vi "LabView - LineFollower.vi"() -> ()   [LabVIEW 2022 SP3]
uses:
  <vilib>/MakerHub/LINX/Public/Peripherals/Digital/Digital Read N Chans.vi
  <vilib>/MakerHub/LINX/Public/Peripherals/Digital/Digital Write N Chans.vi
  <vilib>/MakerHub/LINX/Private/Local IO/LinxDigitalRead.vi
  <vilib>/MakerHub/LINX/Public/Utilities/Check Channel.vi
  <vilib>/MakerHub/LINX/Private/Local IO/LinxDigitalWrite.vi
  <vilib>/MakerHub/LINX/Public/Utilities/Open Serial.vi
  <vilib>/MakerHub/LINX/Private/Utilties/Generate Error.vi
  <vilib>/MakerHub/LINX/Public/Peripherals/PWM/PWM Set Duty Cycle N Chans.vi
  <vilib>/MakerHub/LINX/LMH-LINX.lvlib
panel:
  in  "Slider_Case7":dbl(slide) scale=0.0..1.0
  in  "Slider_Case6":dbl(slide) scale=0.0..1.0
  in  "Slider_Case5":dbl(slide) scale=0.0..1.0
  in  "Slider_Case4":dbl(slide) scale=0.0..1.0
  in  "Slider_Case3":dbl(slide) scale=0.0..1.0
  in  "Slider_Case1":dbl(slide) scale=0.0..1.0
  in  "Slider_Case0":dbl(slide) scale=0.0..1.0
  in  "Array_Case7":bool[](array[boolean])
  in  "Array_Case6":bool[](array[boolean])
  in  "Array_Case5":bool[](array[boolean])
  in  "Array_Case4":bool[](array[boolean])
  in  "ArrayArray_Case3":bool[](array[boolean])
  in  "Array_Case2":bool[](array[boolean])
  in  "Array_Case1":bool[](array[boolean])
  in  "Array_Case0":bool[](array[boolean])
  in  "Motor 1":dbl[](array[slide]) scale=0.0..1.0
  in  "DI Channels":u8[](array[numeric])
  in  "PWM Channels":u8[](array[numeric])
  in  "DO Motor Channels":u8[](array[numeric])
  in  "millisecond timer value":u32
  out "number":u32
  out "String":string
  out "Boolean 2":bool
  out "IR LED":bool[](array[boolean])
  in  "stop":bool
  in  "Serial Port":refnum<visa-resource-name>="N/A"
  # "Motor's PWM"
  # "Motor 1"
  # "Motor 2"
  # "Channels Data"
  # "Data Unit"
  # "IR Cases"
  # "IR Cases Motor's Speed"
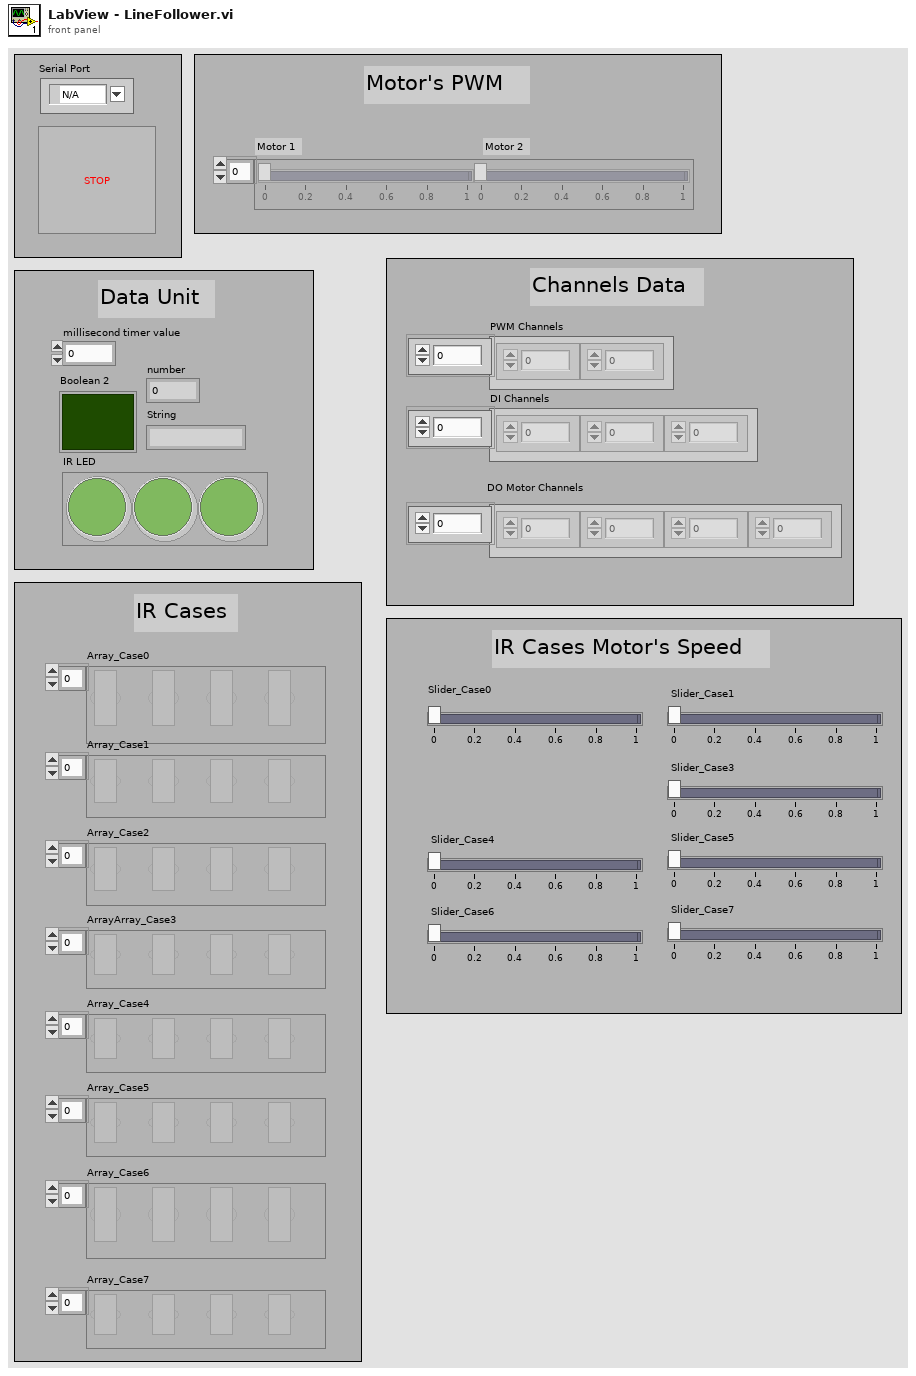
[diagram p1: front panel]
types:
  T1 = typedef "LMH-LINX.lvlib/LINX Ref.ctl" = cluster{"IO":T2, "Interface":T3, "LINX Device Config":T4}
  T2 = typedef "LMH-LINX.lvlib/Platform.ctl" = enum16{"Remote", "Local"}
  T3 = typedef "LMH-LINX.lvlib/Interface.ctl" = enum16{"Serial", "TCP"}
  T4 = typedef "LMH-LINX.lvlib/Device.lvlib/LINX Device Config.ctl" = cluster{"Interface":T3, "COM Port":refnum<visa-resource-name>, "TCP Configuration":T5, "Device Family":u8, "Device ID":u8, "Device Name":string, "TCP Ref":refnum<k5>, "Channels":T6}
  T5 = typedef "LMH-LINX.lvlib/Device.lvlib/TCP Config.ctl" = cluster{"IP Address":string, "Port":u16}
  T6 = typedef "LMH-LINX.lvlib/Channels.ctl" = cluster{"DI":u8[], "DO":u8[], "AI":u8[], "AO":u8[], "PWM":u8[], "QE":u8[], "UART":u8[], "I2C 2":u8[], "SPI":u8[], "CAN":u8[], "Servo":u8[], "AI Ref (V)":dbl, "AI Resolution (Bits)":u8, "AO Ref (V)":dbl, "AO Resolution (Bits)":u8}
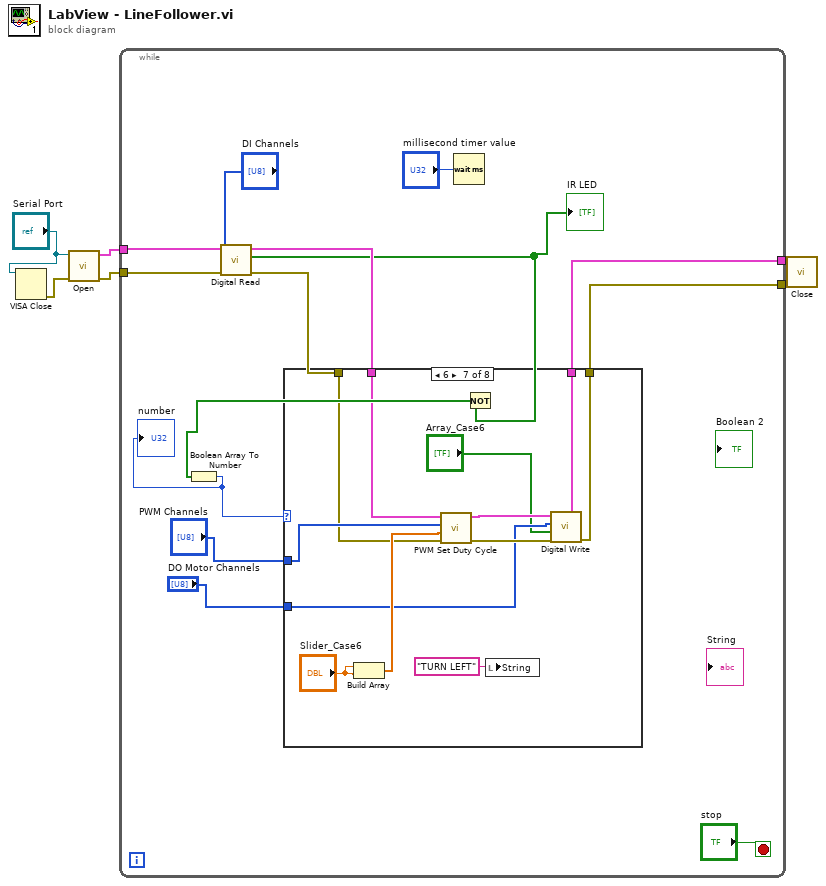
[diagram p0: block diagram]
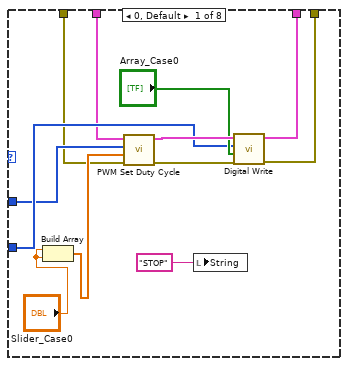
[diagram p2: hidden frame]
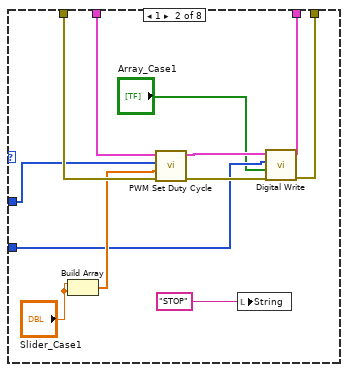
[diagram p3: hidden frame]
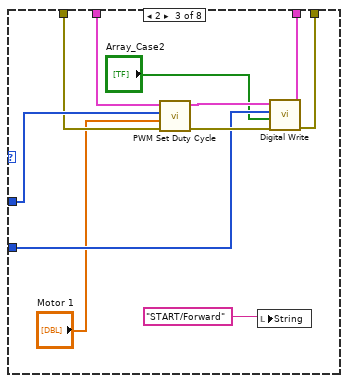
[diagram p4: hidden frame]
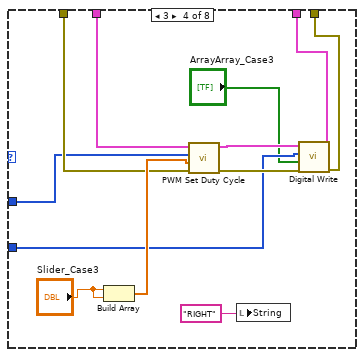
[diagram p5: hidden frame]
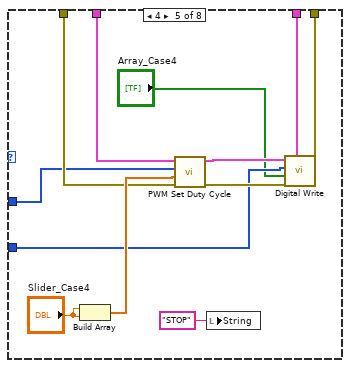
[diagram p6: hidden frame]
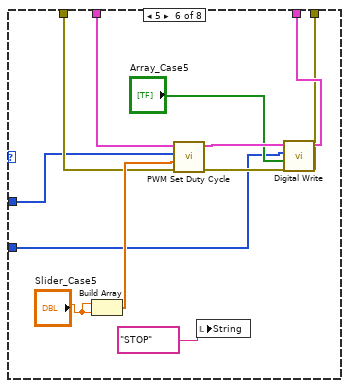
[diagram p7: hidden frame]
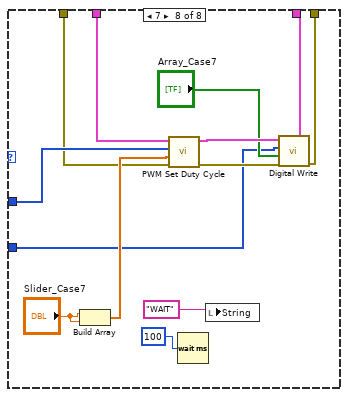
[diagram p8: hidden frame]
diagram:
  n1 = VISA Close(VISA resource name="Serial Port") -> (error out=w5:errorcluster)  [unwired: 1 in]
  n2 = call-poly <vilib>:"Open.vi"("Error In"=w5, "Serial Port"="Serial Port") -> ("Error Out"=w3:errorcluster, "LINX Resource"=w4:T1)  [unwired: 7 in, 1 out]
  n3 = while {
    tunnel: w4 -> [w15]
    tunnel: w3 -> [w14]
    tunnel: [w11] -> w2
    tunnel: [w10] -> w1
    stop <- "stop" stop-if-true
    n4 = call-poly <vilib>:"Digital Read.vi"("Error In"=w14, "DI Channels"="DI Channels", "LINX Resource"=w15) -> ("Error Out"=w12:errorcluster, "Values"=w9:bool[], "LINX Resource"=w13:T1)  [unwired: 6 in]
    "IR LED" <- w9
    n5 = Wait (ms)(milliseconds to wait="millisecond timer value") -> ()  [unwired: 1 out]
    n6 = Not(x=w9) -> (.not. x?=w8:bool[])
    n7 = Boolean Array To Number(Boolean array=w8) -> (number=w18:u32)
    "number" <- w18
    n8 = case shown="6" w18 {
      tunnel: "PWM Channels" -> [w23 w38 w52 w61 w73 w82 w98 w111]
      tunnel: "DO Motor Channels" -> [w27 w37 w51 w60 w72 w81 w99 w108]
      tunnel: [w26 w34 w49 w58 w70 w86 w94 w107] -> w11
      tunnel: [w25 w33 w48 w57 w69 w85 w93 w106] -> w10
      tunnel: w13 -> [w24 w39 w53 w62 w74 w84 w96 w110]
      tunnel: w12 -> [w22 w42 w47 w63 w75 w83 w97 w109]
      frame 0, Default {
        n9 = Build Array("Slider_Case0", "Slider_Case0") -> (w32:dbl[])
        n10 = call-poly <vilib>:"PWM Set Duty Cycle.vi"("Error In"=w22, "Duty Cycles"=w32, "PWM Channels"=w23, "LINX Resource"=w24) -> ("Error Out"=w28:errorcluster, "LINX Resource"=w30:T1)  [unwired: 6 in]
        n11 = local write "String"("STOP") -> ()
        n12 = call-poly <vilib>:"Digital Write.vi"("Error In"=w28, "Values"="Array_Case0", "DO Channels"=w27, "LINX Resource"=w30) -> ("Error Out"=w25:errorcluster, "LINX Resource"=w26:T1)  [unwired: 6 in]
      }
      frame 1 {
        n13 = Build Array("Slider_Case1", "Slider_Case1") -> (w40:dbl[])
        n14 = call-poly <vilib>:"PWM Set Duty Cycle.vi"("Error In"=w42, "Duty Cycles"=w40, "PWM Channels"=w38, "LINX Resource"=w39) -> ("Error Out"=w44:errorcluster, "LINX Resource"=w43:T1)  [unwired: 6 in]
        n15 = local write "String"("STOP") -> ()
        n16 = call-poly <vilib>:"Digital Write.vi"("Error In"=w44, "Values"="Array_Case1", "DO Channels"=w37, "LINX Resource"=w43) -> ("Error Out"=w33:errorcluster, "LINX Resource"=w34:T1)  [unwired: 6 in]
      }
      frame 2 {
        n17 = call-poly <vilib>:"PWM Set Duty Cycle.vi"("Error In"=w47, "Duty Cycles"="Motor 1", "PWM Channels"=w52, "LINX Resource"=w53) -> ("Error Out"=w55:errorcluster, "LINX Resource"=w54:T1)  [unwired: 6 in]
        n18 = local write "String"("START/Forward") -> ()
        n19 = call-poly <vilib>:"Digital Write.vi"("Error In"=w55, "Values"="Array_Case2", "DO Channels"=w51, "LINX Resource"=w54) -> ("Error Out"=w48:errorcluster, "LINX Resource"=w49:T1)  [unwired: 6 in]
      }
      frame 3 {
        n20 = Build Array("Slider_Case3", "Slider_Case3") -> (w64:dbl[])
        n21 = call-poly <vilib>:"PWM Set Duty Cycle.vi"("Error In"=w63, "Duty Cycles"=w64, "PWM Channels"=w61, "LINX Resource"=w62) -> ("Error Out"=w66:errorcluster, "LINX Resource"=w67:T1)  [unwired: 6 in]
        n22 = local write "String"("RIGHT") -> ()
        n23 = call-poly <vilib>:"Digital Write.vi"("Error In"=w66, "Values"="ArrayArray_Case3", "DO Channels"=w60, "LINX Resource"=w67) -> ("Error Out"=w57:errorcluster, "LINX Resource"=w58:T1)  [unwired: 6 in]
      }
      frame 4 {
        n24 = Build Array("Slider_Case4", "Slider_Case4") -> (w76:dbl[])
        n25 = call-poly <vilib>:"PWM Set Duty Cycle.vi"("Error In"=w75, "Duty Cycles"=w76, "PWM Channels"=w73, "LINX Resource"=w74) -> ("Error Out"=w79:errorcluster, "LINX Resource"=w78:T1)  [unwired: 6 in]
        n26 = local write "String"("STOP") -> ()
        n27 = call-poly <vilib>:"Digital Write.vi"("Error In"=w79, "Values"="Array_Case4", "DO Channels"=w72, "LINX Resource"=w78) -> ("Error Out"=w69:errorcluster, "LINX Resource"=w70:T1)  [unwired: 6 in]
      }
      frame 5 {
        n28 = Build Array("Slider_Case5", "Slider_Case5") -> (w88:dbl[])
        n29 = call-poly <vilib>:"PWM Set Duty Cycle.vi"("Error In"=w83, "Duty Cycles"=w88, "PWM Channels"=w82, "LINX Resource"=w84) -> ("Error Out"=w91:errorcluster, "LINX Resource"=w90:T1)  [unwired: 6 in]
        n30 = local write "String"("STOP") -> ()
        n31 = call-poly <vilib>:"Digital Write.vi"("Error In"=w91, "Values"="Array_Case5", "DO Channels"=w81, "LINX Resource"=w90) -> ("Error Out"=w85:errorcluster, "LINX Resource"=w86:T1)  [unwired: 6 in]
      }
      frame 6 {
        n32 = Build Array("Slider_Case6", "Slider_Case6") -> (w100:dbl[])
        n33 = call-poly <vilib>:"PWM Set Duty Cycle.vi"("Error In"=w97, "Duty Cycles"=w100, "PWM Channels"=w98, "LINX Resource"=w96) -> ("Error Out"=w103:errorcluster, "LINX Resource"=w102:T1)  [unwired: 6 in]
        n34 = local write "String"("TURN LEFT") -> ()
        n35 = call-poly <vilib>:"Digital Write.vi"("Error In"=w103, "Values"="Array_Case6", "DO Channels"=w99, "LINX Resource"=w102) -> ("Error Out"=w93:errorcluster, "LINX Resource"=w94:T1)  [unwired: 6 in]
      }
      frame 7 {
        n36 = Build Array("Slider_Case7", "Slider_Case7") -> (w112:dbl[])
        n37 = call-poly <vilib>:"PWM Set Duty Cycle.vi"("Error In"=w109, "Duty Cycles"=w112, "PWM Channels"=w111, "LINX Resource"=w110) -> ("Error Out"=w116:errorcluster, "LINX Resource"=w115:T1)  [unwired: 6 in]
        n38 = Wait (ms)(milliseconds to wait=u32 100 ("millisecond timer value")) -> ()  [unwired: 1 out]
        n39 = local write "String"("WAIT") -> ()
        n40 = call-poly <vilib>:"Digital Write.vi"("Error In"=w116, "Values"="Array_Case7", "DO Channels"=w108, "LINX Resource"=w115) -> ("Error Out"=w106:errorcluster, "LINX Resource"=w107:T1)  [unwired: 6 in]
      }
    }
  }
  n41 = call <vilib>:"Close.vi"("Error In"=w1, "LINX Resource"=w2) -> ()  [unwired: 9 in, 1 out]
